vi "FITS_FormatRecord.vi"(1 "Keyword Value":string, 2 "Keyword Name":string) -> (0 "result string":string)   [LabVIEW 2016]
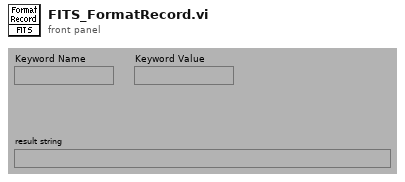
[diagram p1: front panel]
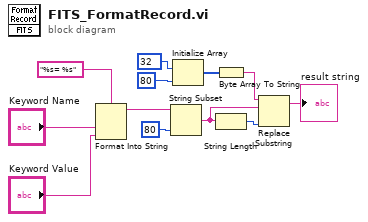
[diagram p0: block diagram]
diagram:
  n1 = Format Into String(format string="%s= %s", "Keyword Name", "Keyword Value") -> (resulting string=w11:string)  [unwired: 2 in, 1 out]
  n2 = String Subset(string=w11, length (rest)=80 ("length (rest)")) -> (substring=w4:string)  [unwired: 1 out]
  n3 = Initialize Array(i8 32 ("Numeric"), 80 ("dimension size")) -> (w7:i8[])
  n4 = Byte Array To String(unsigned byte array=w7) -> (string=w8:string)
  n5 = String Length(string=w4) -> (length=w3:i32)
  n6 = Replace Substring(2:w3, 4:w4, 5:w8) -> (1:→"result string":string)  [unwired: 2 out]
